vi "sub_ekf_observation-model.vi"(11 "x_true":T1) -> (3 "x_true out":T1)   [LabVIEW 2019]
uses:
  <vilib>/Analysis/Matrix/Datatypes/RealMatrix.ctl
  <vilib>/Analysis/baseanly.llb/Real A x B.vi
  <vilib>/Analysis/NI_AALBase.lvlib
  <vilib>/Analysis/Matrix/NI_Matrix.lvlib
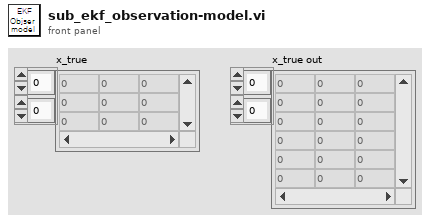
[diagram p1: front panel]
types:
  T1 = typedef "NI_Matrix.lvlib/RealMatrix.ctl" = dbl[][]
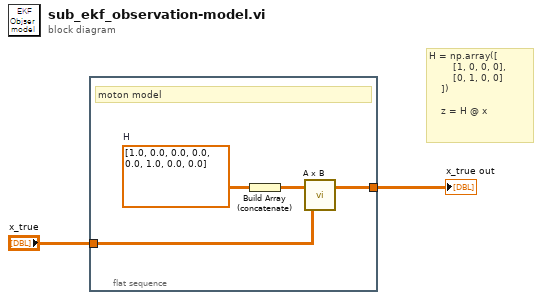
[diagram p0: block diagram]
diagram:
  # "H = np.array([\n        [1, 0, 0, 0],\n        [0, 1, 0, 0]\n    ])\n\n    z = H @ x"
  n1 = flat-sequence {
    tunnel: "x_true" -> [w4]
    tunnel: [w3] -> w1
    frame #0 {
      w6 = dbl[][] [[1.0, 0.0, 0.0, 0.0], [0.0, 1.0, 0.0, 0.0]]  # H
      # "moton model"
      n2 = Build Array (concatenate)(w6) -> (w5:T1)
      n3 = call-poly <vilib>:"A x B.vi"("B"=w4, "A"=w5) -> ("A x B"=w3:T1)  [unwired: 1 out]
    }
  }
  "x_true out" <- w1
